vi "DAQmx Create Channel (CI-Two Edge Separation).vi"(0 "task in":refnum<k21>, 1 "maximum value":dbl=1.0 format="%0.6f", 2 "minimum value":dbl=1e-06 format="%0.6f", 5 "counter":tag, 7 "name to assign":string, 9 "units":i32(ring)=10364 items=["Seconds"=10364, "Ticks"=10304, "From Custom Scale"=10065], 11 "error in":errorcluster, 12 "custom scale name":tag, 13 "first edge":i32(ring)=10280 items=["Rising"=10280, "Falling"=10171], 14 "second edge":i32(ring)=10171 items=["Rising"=10280, "Falling"=10171]) -> (4 "task out":refnum<k21>, 15 "error out":errorcluster)   [LabVIEW 2018]
doc: "Creates a channel that measures the amount of time between the rising or falling edge of one digital signal and the rising or falling edge of another digital signal. With the exception of devices that support multi-counter tasks, you can create only one counter input channel at a time with this VI because a task can contain only one counter input channel. To read from multiple counters simultaneously, use a separate task for each counter. Connect the input signals to the default input terminals of the counter unless you select different input terminals."
uses:
  nilvaiu.dll
panel:
  # "input limits"
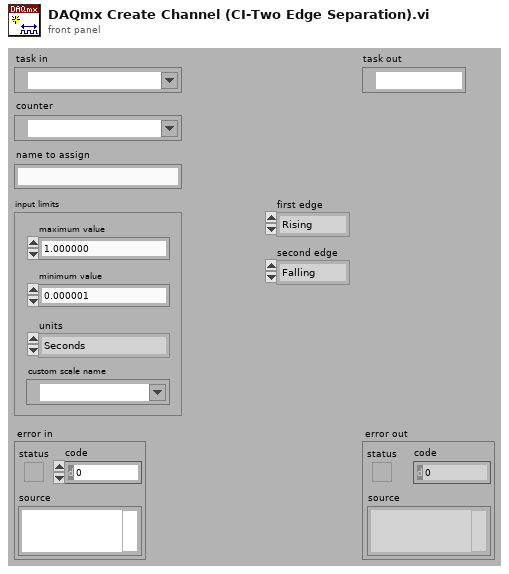
[diagram p1: front panel]
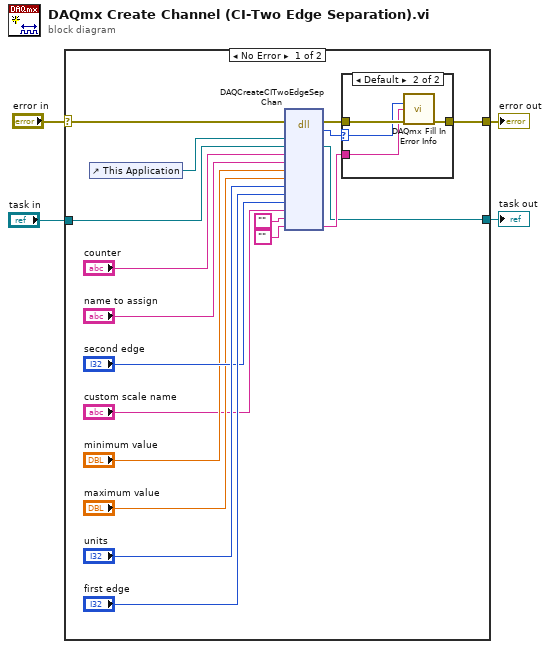
[diagram p0: block diagram]
diagram:
  n1 = case shown="No Error" "error in" {
    selector: "error in" -> [w6 w29]
    tunnel: "task in" -> [w9 w28]
    tunnel: [w8 w28] -> w3
    tunnel: [w7 w29] -> w2
    frame No Error {
      n2 = control-ref of="This Application"() -> (w19:refnum<vi>)
      n3 = dll-call lib="nilvaiu.*" fn="DAQCreateCITwoEdgeSepChan"(error in=w6, "lvAppRef"=w19, "refObjPtr"=w9, "counter"="counter", "channelNameIn"="name to assign", "minVal"="minimum value", "maxVal"="maximum value", "units"="units", "firstEdge"="first edge", "secondEdge"="second edge", "customScaleName"="custom scale name", "channelNamesOut"="", "extendedErrorInfo"="") -> (error out=w22:errorcluster, "return type"=w21:i32, "refObjPtr"=w8:refnum<k21>, "extendedErrorInfo"=w20:string)  [unwired: 12 in, 1 out]
      n4 = case shown="Default" w21 {
        selector: w21 -> [_ w25]
        tunnel: w22 -> [w23 w27]
        tunnel: [w23 w26] -> w7
        tunnel: w20 -> [_ w24]
        frame 0 {
        }
        frame Default {
          n5 = call "DAQmx Fill In Error Info.vi"("status code"=w25, "extended error info"=w24, "error in"=w27) -> ("error out"=w26:errorcluster)  [unwired: 1 in, 11 out]
        }
      }
    }
    frame Error {
    }
  }
  "error out" <- w2
  "task out" <- w3
